vi "DUAL GAUGE-Point -- Terminator.vi"(1 "Eingangstring":string="  0F 400  EE2") -> (0 "Ausgangstring":string="03")   [LabVIEW 2010, in "Dual Gauge.lvlib"]
uses:
  Dual Gauge.lvlib
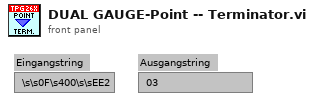
[diagram p1: front panel]
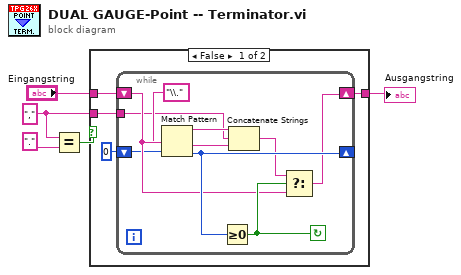
[diagram p0: block diagram]
diagram:
  w1 = "," ("Terminator")
  n1 = Equal?(x=w1, y=".") -> (x = y?=w2:bool)
  n2 = case shown="False" w2 {
    tunnel: [w9 w20] -> w4
    tunnel: "Eingangstring" -> [w7 w20]
    tunnel: w1 -> [w6 _]
    frame False {
      n3 = while {
        tunnel: w6 -> [w10]
        shift-left: w7 -> [w14]
        shift-right: [w13] -> w9
        shift-left: 0 -> [w12]
        shift-right: [w17] -> _
        stop <- w15 continue-if-true
        n4 = Match Pattern(string=w14, regular expression="\\.", offset (0)=w12) -> (before substring=w19:string, after substring=w18:string, offset past match=w17:i32)  [unwired: 1 out]
        n5 = Greater Or Equal To 0?(x=w17) -> (x >= 0?=w15:bool)
        n6 = Concatenate Strings(w19, w10, w18) -> (w16:string)
        n7 = Select(t=w16, s=w15, f=w14) -> (s? t:f=w13:string)
      }
    }
    frame True {
    }
  }
  "Ausgangstring" <- w4
